vi "Get Server Internal UEs.vi"(11 "OOP Server in":refnum<class "Streamer_server.lvclass">) -> (2 "Server Internal UEs":T1, 3 "OOP Server out":refnum<class "Streamer_server.lvclass">)   [LabVIEW 2019, in "Streamer_server.lvlib" / "Streamer_server.lvclass"]
uses:
  Streamer_server.lvclass
  typeDefs/Server Internal UEs.ctl
  typeDefs/Server Internal Message.ctl
  Streamer_server.lvclass/Streamer_server.ctl
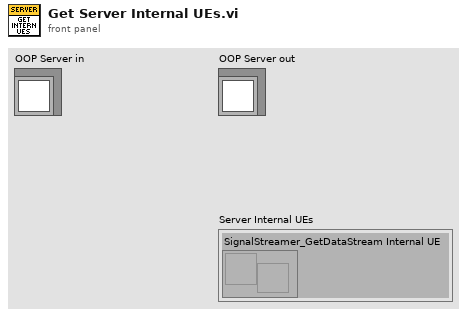
[diagram p1: front panel]
types:
  T1 = typedef "Streamer_server.lvlib/Streamer_server.lvclass/Server Internal UEs.ctl" = cluster{"SignalStreamer_GetDataStream Internal UE":refnum<user-event>}
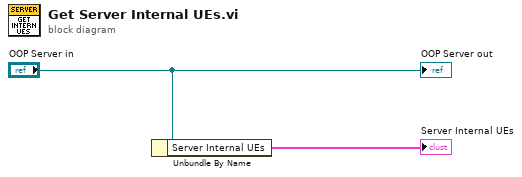
[diagram p0: block diagram]
diagram:
  n1 = Unbundle By Name("OOP Server in") -> ("Server Internal UEs"=→"Server Internal UEs":T1)
  "OOP Server out" <- "OOP Server in"
